vi "LaserCal-Load Data (I-O).vi"(0 "Path":path, 11 "error in (no error)":errorcluster) -> (3 "Stimulus":T4, 4 "I-O Data (static)":T7, 6 "cal type":string, 8 "I-O Data (dynamic)":T2, 10 "Taverage (ms)":dbl, 13 "I-O Data":T1, 14 "Response params":T3, 15 "error out":errorcluster)   [LabVIEW 2020]
uses:
  Typedefs/LaserCal-Data (I-O).ctl
  Typedefs/LaserCal-System ID.ctl
  Typedefs/LaserCal-Stimulus Params.ctl
  Typedefs/LaserCal-Control Mode.ctl
  Typedefs/LaserCal-IO Response Params.ctl
  Typedefs/LaserCal-Data (Dynamic).ctl
  Typedefs/LaserCal-Data (PT).ctl
  <vilib>/Utility/config.llb/Read Key (Double).vi
  epl-vi-lib/Utility VIs/Array Manipulation VIs/Array-Dimensions (2D).vi
  <vilib>/regexp/Match Regular Expression.xnode
  <vilib>/Utility/config.llb/NI_LVConfig.lvlib
panel:
  out "System ID":T6
  out "Info":T8
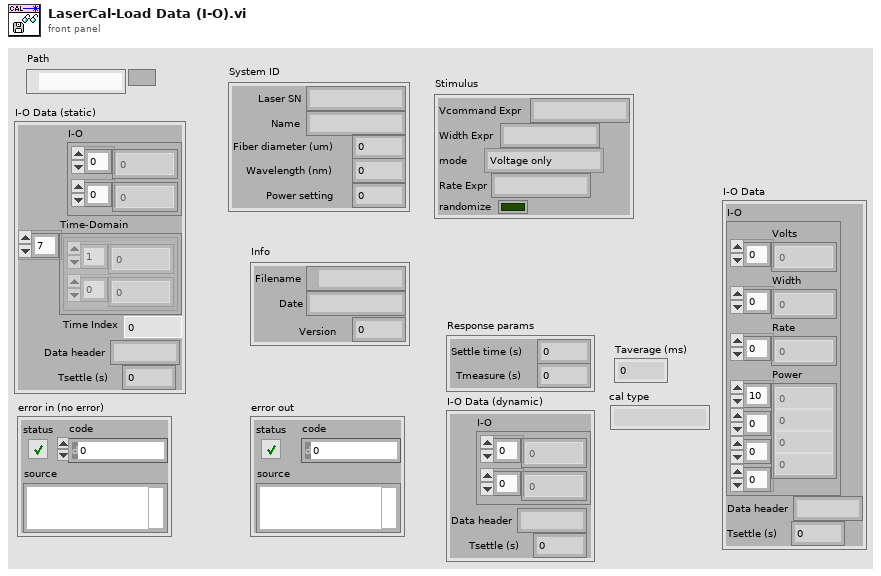
[diagram p1: front panel]
types:
  T1 = typedef "LaserCal-Data (PT).ctl" = cluster{"I-O":cluster{"Volts":dbl[], "Width":dbl[], "Rate":dbl[], "Power":dbl[][][][]}, "Data header":string, "Tsettle (s)":dbl}
  T2 = typedef "LaserCal-Data (Dynamic).ctl" = cluster{"I-O":cluster{dbl[], dbl[]}, "Data header":string, "Tsettle (s)":dbl}
  T3 = typedef "LaserCal-IO Response Params.ctl" = cluster{"Settle time (s)":dbl, "Tmeasure (s)":dbl}
  T4 = typedef "LaserCal-Stimulus Params.ctl" = cluster{"Vcommand Expr":string, "Width Expr":string, "mode":T5, "Rate Expr":string, "randomize":bool}
  T5 = typedef "LaserCal-Control Mode.ctl" = enum16{"Voltage only", "Voltage + Enable"}
  T6 = typedef "LaserCal-System ID.ctl" = cluster{"Name":string, "Laser SN":string, "Wavelength (nm)":dbl, "Fiber diameter (um)":dbl, "Power setting":dbl}
  T7 = typedef "LaserCal-Data (I-O).ctl" = cluster{"I-O":cluster{dbl[], dbl[]}, "Time-Domain":cluster{dbl[], dbl[]}[], "Time Index":i32, "Data header":string, "Tsettle (s)":dbl}
  T8 = cluster{"Filename":path, "Date":string, "Version":i32}
  T9 = typedef "NI_LVConfig.lvlib/Config Data RefNum.ctl" = refnum<k1>
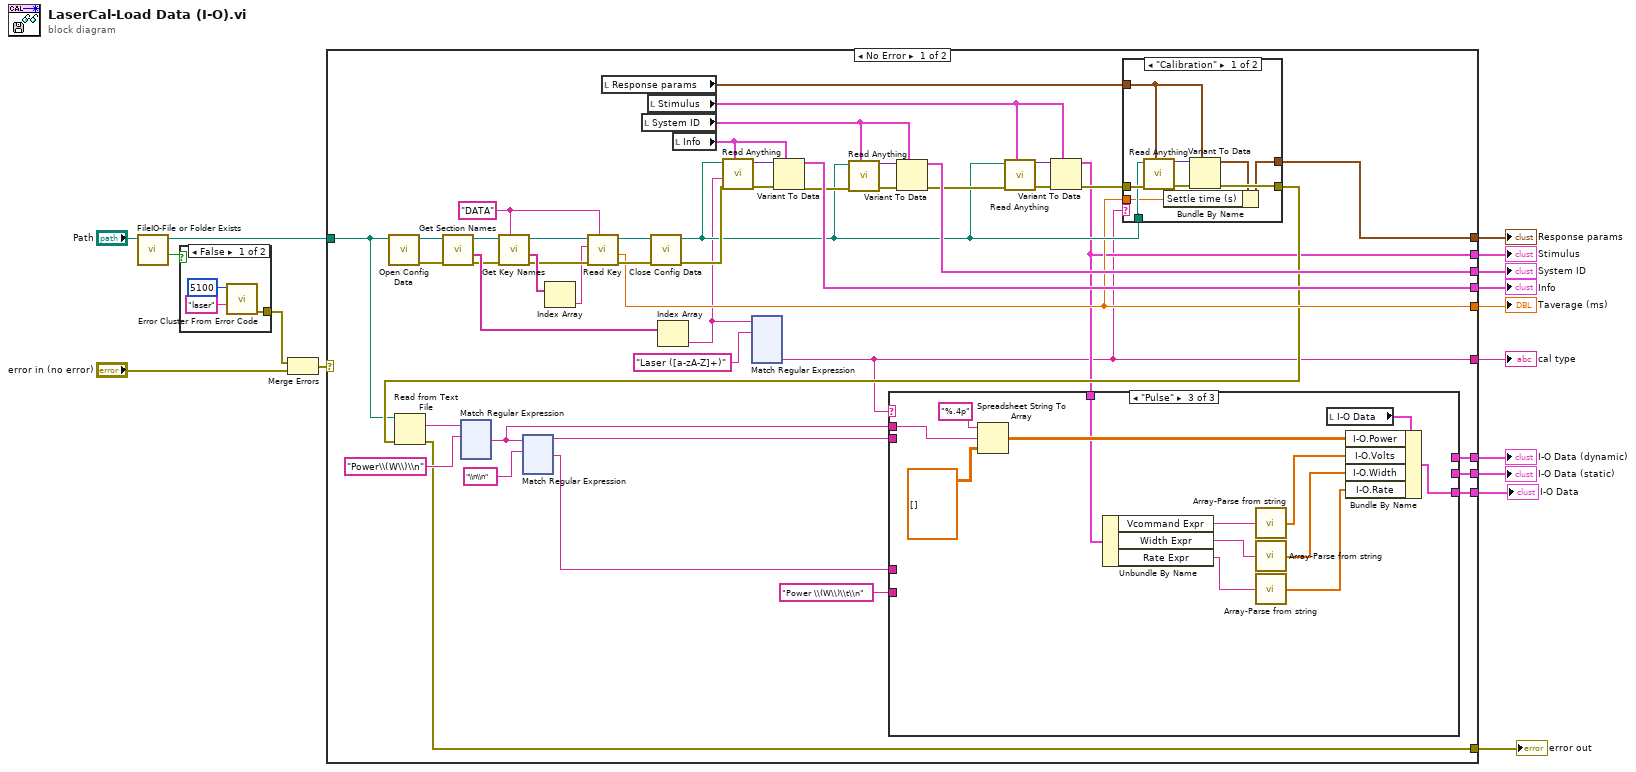
[diagram p0: block diagram]
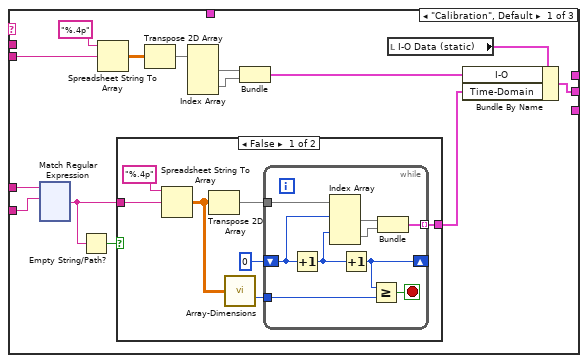
[diagram p3: hidden frame]
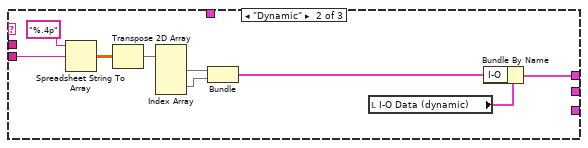
[diagram p5: hidden frame]
diagram:
  n1 = call "FileIO-File or Folder Exists.vi"("path"="Path") -> ("Exists?"=w3:bool, "dup path"=w5:path)  [unwired: 7 in, 2 out]
  n2 = case shown="False" w3 {
    tunnel: [w19 _] -> w1
    frame False {
      n3 = call <vilib>:"Error Cluster From Error Code.vi"("error message (\"\")"="laser" ("error message (\"\")"), "error code (0)"=5100) -> ("error out"=w19:errorcluster)  [unwired: 7 in]
    }
    frame True {
    }
  }
  n4 = Merge Errors(w1, "error in (no error)") -> (w2:errorcluster)
  n5 = case shown="No Error" w2 {
    selector: w2 -> [_ w576]
    tunnel: [w29 w576] -> w16
    tunnel: [w60 _] -> w15
    tunnel: [w55 _] -> w14
    tunnel: [w23 _] -> w13
    tunnel: [w22 _] -> w12
    tunnel: [w47 _] -> w11
    tunnel: [w37 _] -> w10
    tunnel: [w32 _] -> w9
    tunnel: [w31 _] -> w8
    tunnel: [w24 _] -> w7
    tunnel: w5 -> [w20 _]
    frame No Error {
      w41 = "DATA" ("section")
      n6 = call <vilib>:"Open Config Data.vi"("configuration file path"=w20) -> ("error out"=w67:errorcluster, "refnum"=w66:T9)  [unwired: 8 in, 1 out]
      n7 = call <vilib>:"Get Section Names.vi"("error in (no error)"=w67, "refnum"=w66) -> ("error out"=w46:errorcluster, "section names"=w65:string[], "refnum out"=w45:T9)  [unwired: 7 in]
      n8 = call <vilib>:"Get Key Names.vi"("section"=w41, "error in (no error)"=w46, "refnum"=w45) -> ("error out"=w43:errorcluster, "key names"=w44:string[], "refnum out"=w42:T9)  [unwired: 5 in, 1 out]
      n9 = Index Array(array=w44) -> (element=w40:string)  [unwired: 1 in]
      n10 = call-poly <vilib>:"Read Key.vi"("section"=w41, "error in (no error)"=w43, "key"=w40, "refnum"=w42) -> ("error out"=w39:errorcluster, "value"=w37:dbl, "refnum out"=w38:T9)  [unwired: 4 in, 1 out]
      n11 = local read "Response params"() -> (w49:T3)
      n12 = local read "System ID"() -> (w56:T6)
      n13 = local read "Stimulus"() -> (w52:T4)
      n14 = call <vilib>:"Close Config Data.vi"("error in (no error)"=w39, "refnum"=w38) -> ("error out"=w64:errorcluster, "file path"=w48:path)  [unwired: 8 in]
      n15 = Index Array(array=w65) -> (element=w26:string)  [unwired: 1 in]
      n16 = local read "Info"() -> (w61:T8)
      n17 = call "Read Anything.vi"("Type of Anything"=w61, "Error In"=w64, "Section Name (Name of \"Type of Anything\")"=w26, "Path (dialog)"=w48) -> ("Error Out"=w63:errorcluster, "Anything"=w62:variant)  [unwired: 5 in, 1 out]
      n18 = xnode "Match Regular Expression"("input string"=w26, "regular expression"="Laser ([a-zA-Z]+)") -> ("submatch 1"=w22:string)  [unwired: 4 in, 5 out]
      n19 = Variant To Data(error in=w63, type=w61, Variant=w62) -> (data=w60:T8, error out=w59:errorcluster)
      n20 = call "Read Anything.vi"("Type of Anything"=w56, "Error In"=w59, "Path (dialog)"=w48) -> ("Error Out"=w58:errorcluster, "Anything"=w57:variant)  [unwired: 6 in, 1 out]
      n21 = Variant To Data(error in=w58, type=w56, Variant=w57) -> (data=w55:T6, error out=w53:errorcluster)
      n22 = call "Read Anything.vi"("Type of Anything"=w52, "Error In"=w53, "Path (dialog)"=w48) -> ("Error Out"=w51:errorcluster, "Anything"=w54:variant)  [unwired: 6 in, 1 out]
      n23 = Variant To Data(error in=w51, type=w52, Variant=w54) -> (data=w23:T4, error out=w50:errorcluster)
      n24 = case shown="\"Calibration\"" w22 {
        tunnel: w50 -> [w572 w575]
        tunnel: w49 -> [w571 _]
        tunnel: w48 -> [w570 _]
        tunnel: [w569 w575] -> w36
        tunnel: [w567 _] -> w47
        tunnel: w37 -> [w566 _]
        frame "Calibration" {
          n25 = call "Read Anything.vi"("Type of Anything"=w571, "Error In"=w572, "Path (dialog)"=w570) -> ("Error Out"=w573:errorcluster, "Anything"=w574:variant)  [unwired: 6 in, 1 out]
          n26 = Variant To Data(error in=w573, type=w571, Variant=w574) -> (data=w568:T3, error out=w569:errorcluster)
          n27 = Bundle By Name(cluster=w568, "Settle time (s)"=w566) -> (w567:T3)
        }
        frame "Dynamic", Default {
        }
      }
      n28 = Read from Text File(file (use dialog)=w20, error in=w36) -> (text=w35:string, error out=w29:errorcluster)  [unwired: 2 in, 2 out]
      n29 = xnode "Match Regular Expression"("input string"=w35, "regular expression"="Power\\(W\\)\\n") -> ("after match"=w21:string)  [unwired: 4 in, 4 out]
      n30 = xnode "Match Regular Expression"("input string"=w21, "regular expression"="\\n\\n") -> ("before match"=w25:string, "after match"=w30:string)  [unwired: 4 in, 3 out]
      n31 = case shown="\"Pulse\"" w22 {
        tunnel: [_ w330 _] -> w32
        tunnel: [w194 _ _] -> w31
        tunnel: w30 -> [w193 _ _]
        tunnel: "Power \\(W\\)\\t\\n" ("regular expression") -> [w191 _ _]
        tunnel: w25 -> [w182 w322 _]
        tunnel: [_ _ w341] -> w24
        tunnel: w23 -> [_ _ w338]
        tunnel: w21 -> [_ _ w331]
        frame "Calibration", Default {
          n32 = xnode "Match Regular Expression"("input string"=w193, "regular expression"=w191) -> ("after match"=w189:string)  [unwired: 4 in, 4 out]
          n33 = Empty String/Path?(string/path=w189) -> (empty?=w190:bool)
          n34 = Spreadsheet String To Array(format string="%.4p", spreadsheet string=w182) -> (array=w185:dbl[][])  [unwired: 2 in]
          n35 = case shown="False" w190 {
            tunnel: w189 -> [w200 _]
            tunnel: [w197 _] -> w192
            frame False {
              n36 = Spreadsheet String To Array(format string="%.4p", spreadsheet string=w200) -> (array=w195:dbl[][])  [unwired: 2 in]
              n37 = Transpose 2D Array(2D array=w195) -> (transposed array=w199:dbl[][])
              n38 = call-poly "Array-Dimensions.vi"("2D Array"=w195) -> ("# columns"=w196:i32)  [unwired: 13 in, 1 out]
              n39 = while {
                tunnel: w199 -> [w210]
                shift-right: [w203] -> _
                shift-left: 0 -> [w209]
                tunnel: [w205] -> w197 mode=indexing
                tunnel: w196 -> [w202]
                stop <- w204 stop-if-true
                n40 = Increment(x=w209) -> (x+1=w208:i32)
                n41 = Index Array(array=w210, index (row) #1=w209, index (row) #2=w208) -> (element #1=w207:dbl[], element #2=w206:dbl[])  [unwired: 2 in]
                n42 = Increment(x=w208) -> (x+1=w203:i32)
                n43 = Greater Or Equal?(x=w203, y=w202) -> (x >= y?=w204:bool)
                n44 = Bundle(w207, w206) -> (w205:cluster{dbl[], dbl[]})  [unwired: 1 in]
              }
            }
            frame True {
            }
          }
          n45 = Transpose 2D Array(2D array=w185) -> (transposed array=w186:dbl[][])
          n46 = Index Array(array=w186) -> (element #1=w187:dbl[], element #2=w188:dbl[])  [unwired: 4 in]
          n47 = Bundle(w187, w188) -> (w183:cluster{dbl[], dbl[]})  [unwired: 1 in]
          n48 = local read "I-O Data (static)"() -> (w181:T7)
          n49 = Bundle By Name(cluster=w181, "I-O"=w183, "Time-Domain"=w192) -> (w194:T7)
        }
        frame "Dynamic" {
          n50 = Spreadsheet String To Array(format string="%.4p", spreadsheet string=w322) -> (array=w327:dbl[][])  [unwired: 2 in]
          n51 = Transpose 2D Array(2D array=w327) -> (transposed array=w326:dbl[][])
          n52 = Index Array(array=w326) -> (element #1=w325:dbl[], element #2=w324:dbl[])  [unwired: 4 in]
          n53 = Bundle(w325, w324) -> (w323:cluster{dbl[], dbl[]})  [unwired: 1 in]
          n54 = local read "I-O Data (dynamic)"() -> (w329:T2)
          n55 = Bundle By Name(cluster=w329, "I-O"=w323) -> (w330:T2)
        }
        frame "Pulse" {
          n56 = Spreadsheet String To Array(format string="%.4p", spreadsheet string=w331, array type (2D Dbl)=dbl[][][][] []) -> (array=w339:dbl[][][][])  [unwired: 1 in]
          n57 = Unbundle By Name(w338) -> ("Vcommand Expr"=w337:string, "Width Expr"=w335:string, "Rate Expr"=w333:string)
          n58 = call "Array-Parse from string.vi"("String"=w337) -> ("Array"=w336:dbl[])  [unwired: 13 in, 1 out]
          n59 = call "Array-Parse from string.vi"("String"=w335) -> ("Array"=w334:dbl[])  [unwired: 13 in, 1 out]
          n60 = call "Array-Parse from string.vi"("String"=w333) -> ("Array"=w332:dbl[])  [unwired: 13 in, 1 out]
          n61 = local read "I-O Data"() -> (w342:T1)
          n62 = Bundle By Name(cluster=w342, "I-O.Power"=w339, "I-O.Volts"=w336, "I-O.Width"=w334, "I-O.Rate"=w332) -> (w341:T1)
        }
      }
    }
    frame Error {
    }
  }
  "error out" <- w16
  "Info" <- w15
  "I-O Data (static)" <- w8
  "System ID" <- w14
  "Stimulus" <- w13
  "cal type" <- w12
  "Response params" <- w11
  "Taverage (ms)" <- w10
  "I-O Data (dynamic)" <- w9
  "I-O Data" <- w7
